vi "Lian_Lab03_I_Scale_Data.vi"(8 "Boolean":bool, 10 "Scale Factor":dbl, 11 "Input Array":dbl[](array[numeric])) -> (3 "Output Array":dbl[](array[numeric]))   [LabVIEW 2020]
doc: "Receives numeric array and scales elements if Boolean input is True. Otherwise, data flows unchanged."
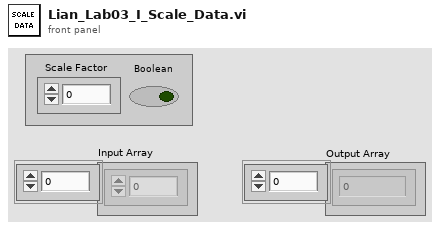
[diagram p1: front panel]
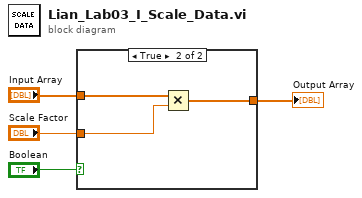
[diagram p0: block diagram]
diagram:
  n1 = case shown="True" "Boolean" {
    tunnel: [w5 w8] -> w1
    tunnel: "Input Array" -> [w5 w7]
    tunnel: "Scale Factor" -> [_ w6]
    frame False {
    }
    frame True {
      n2 = Multiply(x=w7, y=w6) -> (x*y=w8:dbl[])
    }
  }
  "Output Array" <- w1
